vi "Measurement.Init.vi"(8 "error in (no error)":errorcluster, 10 "timeout (5000 ms)":i32=5000, 11 "Measurement.IVCurve in":refnum<class "Measurement.IVCurve.lvclass">) -> (0 "error out":errorcluster, 1 "Dependencies Results":bool[](array[boolean]), 2 "Result":bool, 3 "Measurement.IVCurve out":refnum<class "Measurement.IVCurve.lvclass">)   [LabVIEW 2019, in "Measurement.IVCurve.lvclass"]
uses:
  Measurement.IVCurve.lvclass
  SMU/SMU.lvclass
  E:/UPWORK/Laser Tool/Laser/project/Subsystems/Device/Device.lvclass
  Device/Device.lvclass
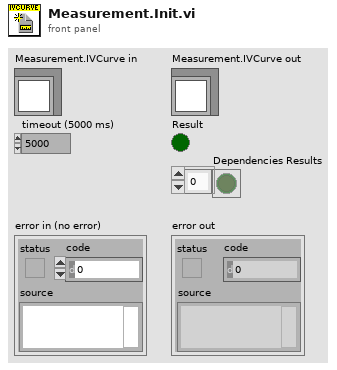
[diagram p1: front panel]
types:
  T1 = typedef "Measurement.IVCurve.lvclass/Configuration--Cluster.ctl" = cluster{"Measurement.Type":T2, "Hardware":T3, "Measurement":T6}
  T2 = typedef "Measurement.lvclass/Measurement.Type--Enum.ctl" = enum16{"Free", "I/V Curve", "Wavelength sweeping", "Photocurrent mapping"}
  T3 = typedef "Measurement.IVCurve.lvclass/Configuration.Hardware--Cluster.ctl" = cluster{"SMU":T4}
  T4 = typedef "Measurement.lvclass/Configuration.SMU--Cluster.ctl" = cluster{"Enable":bool, "SMU Model":string, "Configuration":T5}
  T5 = typedef "SMU.lvclass/Configuration--Cluster.ctl" = cluster{"VISA Resource":string, "Channel":string}
  T6 = typedef "Measurement.IVCurve.lvclass/Configuration.Measurement--Cluster.ctl" = cluster{"SMU Voltage Start, V":dbl, "SMU Voltage Stop, V":dbl, "SMU Voltage Step, V":dbl, "Delay time, ms":u16, "Accumulation":u16}
  T7 = typedef "Measurement.IVCurve.lvclass/Dependencies--Cluster.ctl" = cluster{"SMU":refnum<class "SMU.lvclass">}
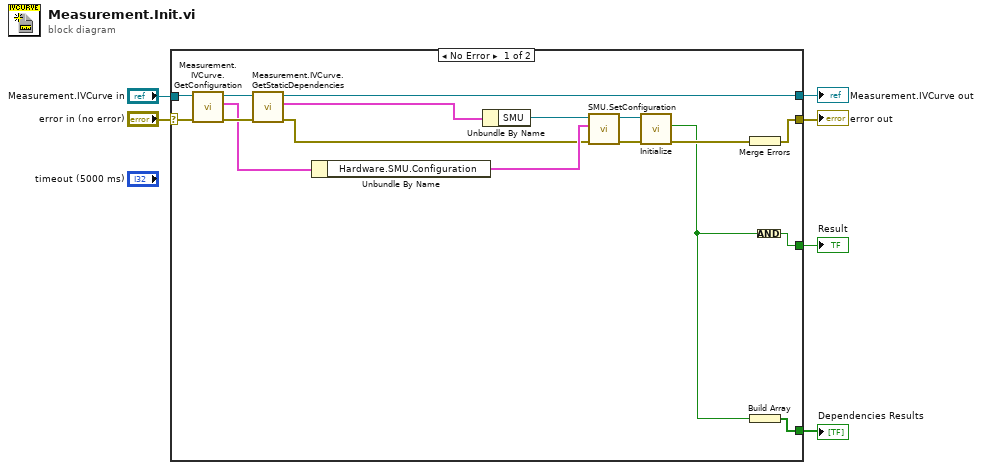
[diagram p0: block diagram]
diagram:
  n1 = case shown="No Error" "error in (no error)" {
    selector: "error in (no error)" -> [w22 w24]
    tunnel: "Measurement.IVCurve in" -> [w23 w25]
    tunnel: [w10 w25] -> w4
    tunnel: [w9 w24] -> w3
    tunnel: [w8 _] -> w1
    tunnel: [w7 _] -> w2
    frame No Error {
      n2 = call "Measurement.IVCurve.GetConfiguration.vi"("error in (no error)"=w22, "Measurement.IVCurve"=w23) -> ("error out"=w20:errorcluster, "Configuration"=w13:T1, "Measurement.IVCurve out"=w21:refnum<class "Measurement.IVCurve.lvclass">)  [unwired: 7 in]
      n3 = call "Measurement.IVCurve.GetStaticDependencies.vi"("error in (no error)"=w20, "Measurement.IVCurve in"=w21) -> ("error out"=w12:errorcluster, "Dependencies"=w11:T7, "Measurement.IVCurve out"=w10:refnum<class "Measurement.IVCurve.lvclass">)  [unwired: 7 in]
      n4 = Unbundle By Name(w13) -> ("Hardware.SMU.Configuration"=w18:T5)
      n5 = Unbundle By Name(w11) -> ("SMU"=w19:refnum<class "SMU.lvclass">)
      n6 = call "SMU.SetConfiguration.vi"("error in (no error)"=w12, "Configuration"=w18, "SMU"=w19) -> ("error out"=w16:errorcluster, "SMU out"=w17:refnum<class "SMU.lvclass">)  [unwired: 7 in]
      n7 = call "Initialize.vi"("error in (no error)"=w16, "Device in"=w17) -> ("error out"=w15:errorcluster, "Result"=w14:bool)  [unwired: 7 in, 1 out]
      n8 = Merge Errors(w15) -> (w9:errorcluster)
      n9 = Build Array(w14) -> (w7:bool[])
      n10 = Compound Arithmetic op=AND(w14) -> (w8:bool)
    }
    frame Error {
    }
  }
  "error out" <- w3
  "Measurement.IVCurve out" <- w4
  "Result" <- w1
  "Dependencies Results" <- w2
